vi "ziGetValueDIO.vi"(3 "error in":errorcluster, 5 "Path":string, 6 "Handle In":T1 {"Handle" format="0x%08x"; "Conn" format="0x%08x"}) -> (0 "error out":errorcluster, 1 "DIO Value":cluster{"dt (ticks)":u64, "value":u32}, 2 "Handle Out":T1 {"Handle" format="0x%08x"; "Conn" format="0x%08x"})   [LabVIEW 2009, in "Zurich Instruments LabOne.lvlib"]
doc: "This vi retrieves the newest available DIO sample from the specified node. The vi returns the value first found if more than one value is available (a wildcard is used in the Path). This function is only applicable to nodes ending in \"DIOS/[0-9]+/input\"."
uses:
  <instrlib>/Zurich Instruments LabOne/Zurich Instruments LabOne.lvlib
  <instrlib>/Zurich Instruments LabOne/Public/ziTypeHandle.ctl
  <instrlib>/Zurich Instruments LabOne/Private/ziLV32.dll
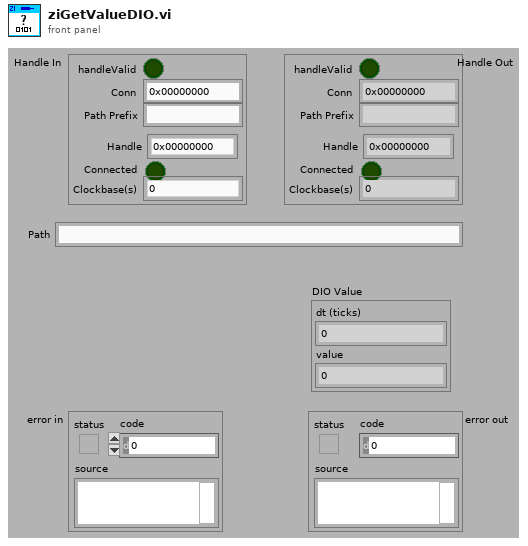
[diagram p1: front panel]
types:
  T1 = typedef "Zurich Instruments LabOne.lvlib/ziTypeHandle.ctl" = cluster{"handleValid":bool, "Conn":u64, "Path Prefix":string, "Handle":u64, "Connected":bool, "Clockbase(s)":dbl}
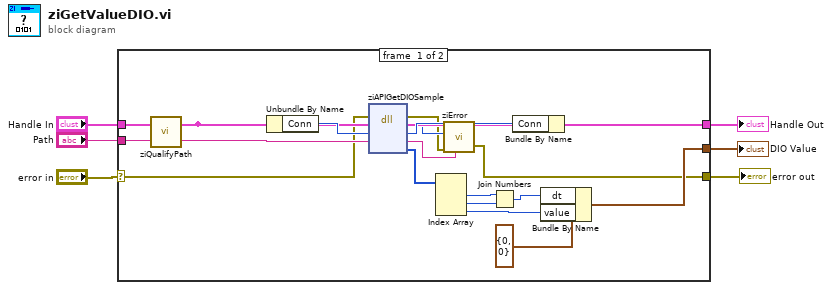
[diagram p0: block diagram]
diagram:
  n1 = case shown="No Error" "error in" {
    selector: "error in" -> [w8 w27]
    tunnel: [w25 w26] -> w6
    tunnel: [w24 _] -> w5
    tunnel: "Path" -> [w14 _]
    tunnel: "Handle In" -> [w13 w26]
    tunnel: [w12 w27] -> w2
    frame #0 {
      n2 = call <instrlib>:"ziQualifyPath.vi"("Path In"=w14, "Handle In"=w13) -> ("Path Out"=w15:string, "Handle Out"=w16:T1)
      n3 = Unbundle By Name(w16) -> ("Conn"=w23:u64)
      n4 = dll-call lib="C:/Program Files (x86)/National Instruments/LabVIEW 2009/instr.lib/Zurich Instruments LabOne/Private/ziLV*.*" fn="ziAPIGetDIOSample" label="ziAPIGetValueDIO"(error in=w8, "Conn"=w23, "Path"=w15) -> (error out=w9:errorcluster, "return type"=w11:u32, "Conn"=w22:u64, "Path"=w7:string, "DIOSample"=w21:u32[])  [unwired: 2 in, 2 out]
      n5 = Index Array(array=w21) -> (element #1=w18:u32, element #2=w17:u32, element #3=w19:u32)  [unwired: 3 in]
      n6 = call <instrlib>:"ziError.vi"("ziErrorCode"=w11, "Error In"=w9, "Annotation"=w7) -> ("Error Out"=w12:errorcluster)  [unwired: 3 in]
      n7 = Join Numbers(hi=w18, lo=w17) -> ((hi.lo)=w10:u64)
      n8 = Bundle By Name(cluster=w16, "Conn"=w22) -> (w25:T1)
      n9 = Bundle By Name(cluster=cluster{"dt":u64, "value":u32} {"dt"=0, "value"=0} ("DioVal"), "dt"=w10, "value"=w19) -> (w24:cluster{"dt":u64, "value":u32})
    }
    frame #1 {
    }
  }
  "Handle Out" <- w6
  "error out" <- w2
  "DIO Value" <- w5
